vi "Write Settings path.vi"(8 "error in (no error)":errorcluster, 10 "Settings path":path, 11 "Load-settings in":refnum<class "Load-settings.lvclass">) -> (0 "error out":errorcluster, 3 "Load-settings out":refnum<class "Load-settings.lvclass">)   [LabVIEW 2013, in "Messages.lvlib" / "Load-settings.lvclass"]
uses:
  Load-settings.lvclass
  Load-settings.lvclass/Load-settings.ctl
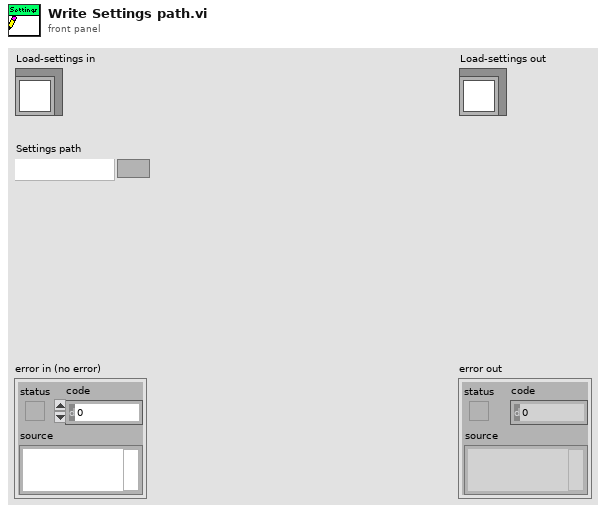
[diagram p1: front panel]
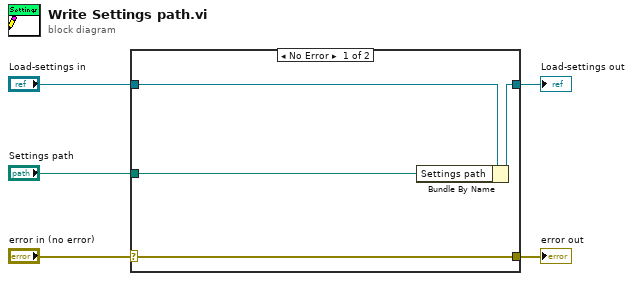
[diagram p0: block diagram]
diagram:
  n1 = case shown="No Error" "error in (no error)" {
    selector: "error in (no error)" -> [w9 w10]
    tunnel: [w9 w10] -> w4
    tunnel: [w7 w11] -> w2
    tunnel: "Load-settings in" -> [w8 w11]
    tunnel: "Settings path" -> [w6 _]
    frame No Error {
      n2 = Bundle By Name(cluster=w8, "Settings path"=w6) -> (w7:refnum<class "Load-settings.lvclass">)
    }
    frame Error {
    }
  }
  "error out" <- w4
  "Load-settings out" <- w2
